vi "Master_DARPA_FUS2.vi"() -> ()   [LabVIEW 2021]
uses:
  Control 2.ctl
  Settings.ctl
  <vilib>/DAQmx/write.llb/DAQmx Write (Analog DBL 1Chan 1Samp).vi
  <vilib>/DAQmx/write.llb/DAQmx Write (Analog Wfm 1Chan NSamp).vi
  <vilib>/DAQmx/write.llb/DAQmx Write (Digital 1D U32 1Chan NSamp).vi
  <vilib>/DAQmx/read.llb/DAQmx Read (Counter DBL 1Chan 1Samp).vi
  <vilib>/DAQmx/create/channels.llb/DAQmx Create Channel (AO-Voltage-Basic).vi
  <vilib>/DAQmx/create/channels.llb/DAQmx Create Channel (CI-Count Edges).vi
  <vilib>/DAQmx/miscellaneous.llb/DAQmx Fill In Error Info.vi
  <vilib>/DAQmx/create/channels.llb/DAQmx Create Channel (DO-Digital Output).vi
  <vilib>/DAQmx/configure/timing.llb/DAQmx Timing (Sample Clock).vi
  <resource>/objmgr/daqmx.rc
panel:
  out "Trial End Signal":bool=TRUE
  in  "stop":bool
  in  "Blue Exposure Width [50-100] (ms)":T1=41.0 format="%#_9f"
  in  "Amber Start Time":T1=60.0 format="%#_9f"
  in  "Red Start (ms)":T1=120.0 format="%#_9f"
  in  "Red Exposure Width (ms)":T1=41.0 format="%#_9f"
  in  "Amber Exposure Width (ms)":T1=41.0 format="%#_9f"
  in  "base path":path=path "E:/DARPA/TUS-LSCI6"
  in  "Delay end (ms)":dbl=102.0
  out "Stimulation":bool=TRUE
  in  "AOM Voltage":dbl=0.085 format="%0.3f"
  out "String 7":string="AOM Settings"
  out "String 6":string="Stroke Settings"
  out "String 5":string="Intrinsic Imaging"
  in  "LED 625 nm":bool
  in  "LED 580 nm":bool
  out "Trial #":i32=6
  out "Frames acquired":dbl=9000.0 format="%0.2f"
  out "Number of Samples (Total)":dbl=18000.0
  out "Period (ms)":dbl=6.5
  out "String 4":string="Experimental Summary"
  out "String 3":string="Stimulation Control"
  out "String 2":string="Sequence Control"
  out "String":string="Trials Control"
  in  "# of stimulations":i32=112
  in  "Width of pulse (ms)":dbl=60.0
  in  "# of Sequences":dbl=750.0
  in  "Sampling Rate (Hz)":T1=100000.0 format="%#_9f"
  in  "Frames/Seq":i32=12
  in  "Exposure Width (ms)":T1=5.0 format="%#_9f"
  in  "Time Between (ms)":T2=1.5 format="%#_9f"
  in  "Pre-stimulus Time":dbl=30.0 format="%.6f"
  in  "Time b/w Trials (s)":dbl=5.0 caption="Delay Time (s)"
  in  "# Trials":i32=6
  in  "Time domain signal":T3(tab)=enum."Stimulation pulse"
  out "LSCI Sequence":cluster{i32, dbl, dbl[]}(graph)={0, 1e-05, array[18000 elements]}
  out "Red LED":cluster{i32, dbl, dbl[]}(graph)={0, 1e-05, array[18000 elements]}
  out "Amber LED":cluster{i32, dbl, dbl[]}(graph)={0, 1e-05, array[18000 elements]}
  out "Blue LED":cluster{i32, dbl, dbl[]}(graph)={0, 1e-05, array[18000 elements]}
  out "EMCCD":cluster{i32, dbl, dbl[]}(graph)={0, 1e-05, array[18000 elements]}
  out "Whisker Cam":cluster{i32, dbl, dbl[]}(graph)={0, 1e-05, array[18000 elements]}
  out "Whisker Stim":cluster{i32, dbl, dbl[]}(graph)={0, 1e-05, array[18000 elements]}
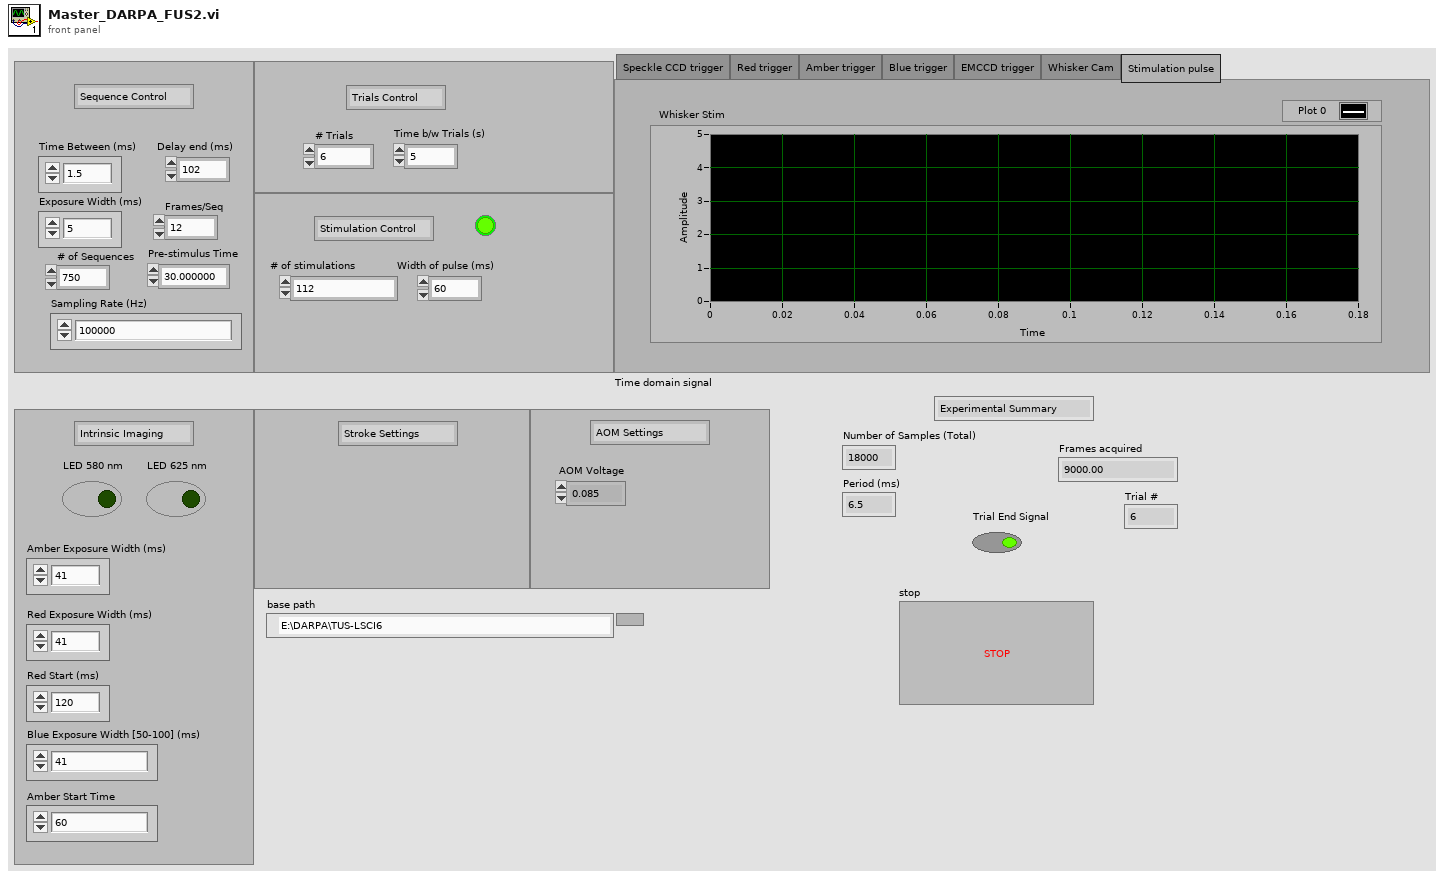
[diagram p1: front panel]
types:
  T1 = typedef "Settings.ctl" = dbl
  T2 = typedef "Control 2.ctl" = dbl
  T3 = enum32{"Speckle CCD trigger", "Red trigger", "Amber trigger", "Blue trigger", "EMCCD trigger", "Whisker Cam", "Stimulation pulse"}
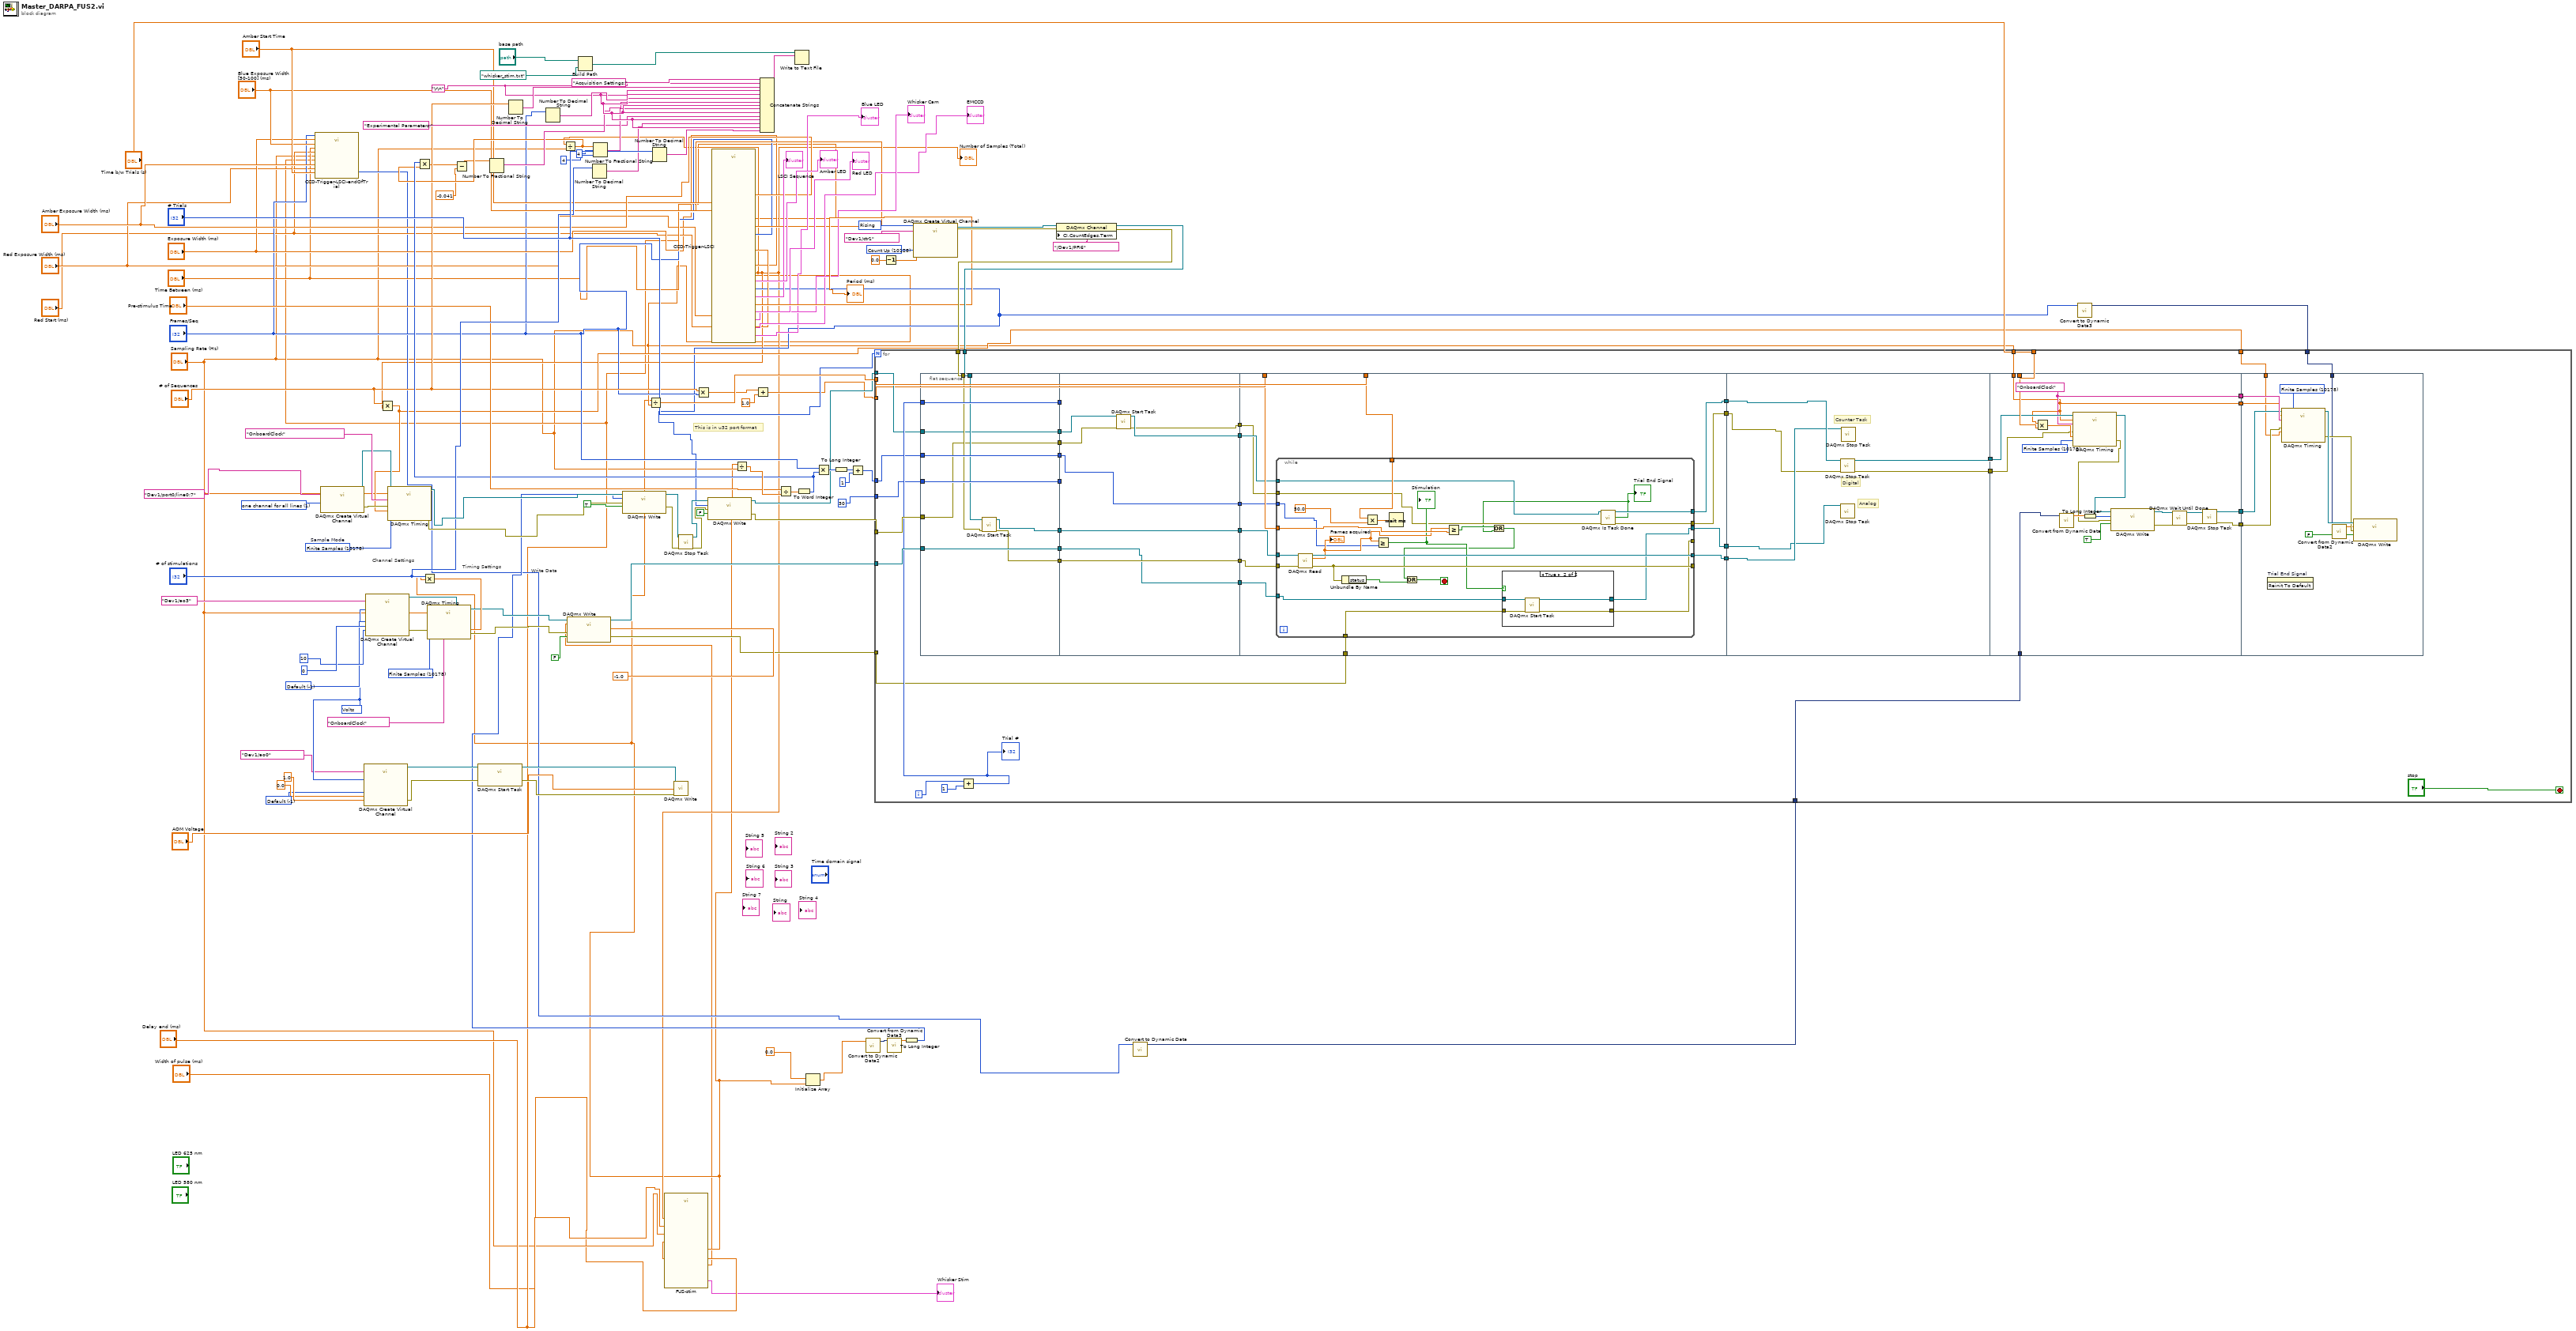
[diagram p0: block diagram]
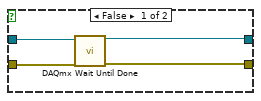
[diagram p2: hidden frame]
diagram:
  w64 = "\r\n"
  w74 = 1 items=["one channel for each line", "one channel for all lines"] ("line grouping")
  w89 = -1 items=["Default"=-1, "RSE"=10083, "Differential"=10106, "Pseudodifferential"=12529] ("output terminal configuration")
  w99 = 10280 items=["Rising"=10280, "Falling"=10171] ("edge")
  w103 = 10128 items=["Count Up"=10128, "Count Down"=10124, "Externally Controlled"=10326] ("count direction")
  w113 = 10178 items=["Finite Samples"=10178, "Continuous Samples"=10123] ("sample mode")
  w114 = -1 items=["Default"=-1, "RSE"=10083, "Differential"=10106, "Pseudodifferential"=12529] ("output terminal configuration")
  w91 = 10348 items=["Volts"=10348, "From Custom Scale"=10065] ("units")
  w119 = 10178 items=["Finite Samples"=10178, "Continuous Samples"=10123, "Hardware Timed Single Point"=12522]  # Sample Mode
  # "This is in u32 port format"
  # "Timing Settings"
  # "Write Data"
  # "Channel Settings"
  n1 = call "CCD-Trigger-LSCI-endOfTrial.vi"("Frames/Seq"="Frames/Seq", "Exposure Width (ms) in"="Exposure Width (ms)", "Blue Exposure Width [50-100] (ms)"="Blue Exposure Width [50-100] (ms)", "Time Between (ms)"="Time Between (ms)", "Red Start Time"="Red Start (ms)", "Sampling Rate"="Sampling Rate (Hz)", "Amber Start Time"="Amber Start Time", "Red Exposure Width [50-80] (ms)"="Red Exposure Width (ms)", "Amber Exposure Width [50-100] (ms)"="Amber Exposure Width (ms)", "Delay End (ms)"="Delay end (ms)") -> ("Array out"=w15:u32[])  [unwired: 1 in, 8 out]
  n2 = call-poly <vilib>:"DAQmx Create Virtual Channel.vi"("lines"=tag "Dev1/port0/line0:7", "line grouping"=w74) -> ("task out"=w81:refnum<k21>, "error out"=w107:errorcluster)  [unwired: 12 in]
  n3 = call-poly <vilib>:"DAQmx Create Virtual Channel.vi"("maximum value"=1.0, "minimum value"=0.0, "output terminal configuration"=w89, "physical channels"=tag "Dev1/ao0", "units"=w91) -> ("task out"=w87:refnum<k21>, "error out"=w86:errorcluster)  [unwired: 9 in]
  n4 = call-poly <vilib>:"DAQmx Create Virtual Channel.vi"("maximum value"=10, "minimum value"=0, "output terminal configuration"=w114, "physical channels"=tag "Dev1/ao3", "units"=w91) -> ("task out"=w111:refnum<k21>, "error out"=w112:errorcluster)  [unwired: 9 in]
  n5 = call <vilib>:"DAQmx Start Task.vi"("task/channels in"=w87, "error in"=w86) -> ("task out"=w85:refnum<k21>, "error out"=w84:errorcluster)  [unwired: 12 in]
  n6 = Number To Decimal String(number="# of Sequences") -> (decimal integer string=w66:string)  [unwired: 1 in]
  n7 = Number To Decimal String(number="Frames/Seq") -> (decimal integer string=w65:string)  [unwired: 1 in]
  n8 = Build Path(base path="base path", name or relative path=path "whisker_stim.txt" ("default name")) -> (appended path=w68:path)
  n9 = Number To Decimal String(number="# of stimulations") -> (decimal integer string=w59:string)  [unwired: 1 in]
  n10 = Number To Decimal String(number="# Trials") -> (decimal integer string=w63:string)  [unwired: 1 in]
  n11 = call-poly <vilib>:"DAQmx Write.vi"("task/channels in"=w85, "data"="AOM Voltage", "error in"=w84) -> ()  [unwired: 10 in, 3 out]
  n12 = Multiply(x="# of Sequences", y="Frames/Seq") -> (x*y=w18:dbl)
  n13 = call "CCD-Trigger-LSCI.vi"("Frames/Seq"="Frames/Seq", "Exposure Width (ms) in"="Exposure Width (ms)", "Blue Exposure Width [50-100] (ms)"="Blue Exposure Width [50-100] (ms)", "Time Between (ms)"="Time Between (ms)", "Red Start Time"="Red Start (ms)", "Sampling Rate"="Sampling Rate (Hz)", "Amber Start Time"="Amber Start Time", "Red Exposure Width [50-80] (ms)"="Red Exposure Width (ms)", "Amber Exposure Width [50-100] (ms)"="Amber Exposure Width (ms)", "Delay End (ms)"="Delay end (ms)") -> ("Blue LED"=→"Blue LED":cluster{i32, dbl, dbl[]}, "LSCI CCD"=→"LSCI Sequence":cluster{i32, dbl, dbl[]}, "Amber LED"=→"Amber LED":cluster{i32, dbl, dbl[]}, "Whisker Cam"=→"Whisker Cam":cluster{i32, dbl, dbl[]}, "EMCCD Trigger"=→"EMCCD":cluster{i32, dbl, dbl[]}, "Array out"=w12:u32[], "Period (ms)"=→"Period (ms)":dbl, "# Samples"=w7:T1, "Red LED"=→"Red LED":cluster{i32, dbl, dbl[]})  [unwired: 1 in]
  "Number of Samples (Total)" <- w7
  n14 = Multiply(x="# of Sequences", y=w7) -> (x*y=w13:T1)
  n15 = call-poly <vilib>:"DAQmx Timing.vi"("task/channels in"=w81, "sample mode"=w119, "samples per channel"=w13, "rate"="Sampling Rate (Hz)", "source"=tag "OnboardClock", "error in"=w107) -> ("task out"=w76:refnum<k21>, "error out"=w75:errorcluster)  [unwired: 8 in]
  n16 = Divide(x=w7, y="Sampling Rate (Hz)") -> (x/y=w48:T1)
  n17 = Number To Fractional String(number=w48, width (-)=i16 4, precision (6)=i16 4) -> (F-format string=w58:string)  [unwired: 1 in]
  n18 = call "FUS-stim.vi"("# Samples in"=w7, "Delay end (ms)"="Delay end (ms)", "Width of pulse (ms)"="Width of pulse (ms)", "Sampling Rate"="Sampling Rate (Hz)") -> ("Array 2"=w2:T1[], "# Samples out"=w3:T1, "Stimulation 2"=→"Whisker Stim":cluster{i32, dbl, dbl[]})  [unwired: 3 in, 2 out]
  n19 = Multiply(x="# of stimulations", y=w3) -> (x*y=w108:T1)
  n20 = call-poly <vilib>:"DAQmx Timing.vi"("task/channels in"=w111, "sample mode"=w113, "samples per channel"=w108, "rate"="Sampling Rate (Hz)", "source"=tag "OnboardClock", "error in"=w112) -> ("task out"=w78:refnum<k21>, "error out"=w77:errorcluster)  [unwired: 1 in, 7 out]
  n21 = call-poly <vilib>:"DAQmx Write.vi"("task/channels in"=w78, "auto start"=FALSE, "data"=w2, "timeout"=-1.0 ("Wirite Timeout"), "error in"=w77) -> ("task out"=w82:refnum<k21>, "error out"=w96:errorcluster)  [unwired: 9 out]
  n22 = Divide(x=w3, y="Sampling Rate (Hz)") -> (x/y=w95:T1)
  n23 = Divide(x=w3, y="Sampling Rate (Hz)") -> (x/y=w73:T1)
  n24 = Add(x=w18, y=1.0) -> (x+y=w16:dbl)
  n25 = Divide(x="Pre-stimulus Time", y=w73) -> (x/y=w52:T1)
  n26 = To Word Integer(number=w52) -> (16bit integer=w51:i16)
  n27 = Multiply(x=w51, y=w48) -> (x*y=w9:T1)
  n28 = Subtract(x=w9, y=-0.041) -> (x-y=w10:T1)
  n29 = Number To Fractional String(number=w10) -> (F-format string=w55:string)  [unwired: 3 in]
  n30 = Concatenate Strings("Acquisition Settings:" ("string"), w64, w66, w64, w65, w64, w55, w64, w58, w64, "Experimental Parameters:" ("string"), w64, w59, w64, w63) -> (w62:string)
  n31 = Write to Text File(file (use dialog)=w68, text=w62) -> ()  [unwired: 2 in, 3 out]
  n32 = Initialize Array(0.0 ("element"), w3) -> (w19:dbl[])
  n33 = Multiply(x="Frames/Seq", y=w51) -> (x*y=w53:i32)
  n34 = To Long Integer(number=w53) -> (32bit integer=w47:i32)
  n35 = Add(x=w47, y=1) -> (x+y=w45:i32)
  n36 = call "Convert to Dynamic Data2"("Array"=w19) -> ("Dynamic Data Type"=w37:dynamicdata)  [unwired: 3 in]
  n37 = Decrement(x=0.0) -> (x-1=w102:dbl)
  n38 = call "Convert from Dynamic Data3"("Dynamic Data Type"=w37) -> ("Array"=w36:dbl[])  [unwired: 3 in]
  n39 = To Long Integer(number=w36) -> (32bit integer=w35:i32[])
  n40 = call-poly <vilib>:"DAQmx Write.vi"("task/channels in"=w76, "auto start"=TRUE, "data"=w35, "error in"=w75) -> ("task out"=w31:refnum<k21>, "error out"=w29:errorcluster)  [unwired: 9 in, 1 out]
  n41 = call <vilib>:"DAQmx Stop Task.vi"("task/channels in"=w31, "error in"=w29) -> ("task out"=w30:refnum<k21>, "error out"=w28:errorcluster)  [unwired: 12 in]
  n42 = call-poly <vilib>:"DAQmx Write.vi"("task/channels in"=w30, "auto start"=FALSE, "data"=w12, "error in"=w28) -> ("task out"=w32:refnum<k21>, "error out"=w33:errorcluster)  [unwired: 9 in, 1 out]
  n43 = call-poly <vilib>:"DAQmx Create Virtual Channel.vi"("initial count"=w102, "count direction"=w103, "edge"=w99, "counter"=tag "Dev1/ctr1") -> ("task out"=w100:refnum<k21>, "error out"=w101:errorcluster)  [unwired: 10 in]
  n44 = property class="DAQmx Channel"(reference=w100, error in=w101, "CI.CountEdges.Term"=tag "/Dev1/PFI6") -> (reference out=w71:refnum<k21>, error out=w72:errorcluster)
  n45 = call "Convert to Dynamic Data"("Array"=w15) -> ("Dynamic Data Type"=w14:dynamicdata)  [unwired: 3 in]
  n46 = call "Convert to Dynamic Data3"("Array"=w12) -> ("Dynamic Data Type"=w11:dynamicdata)  [unwired: 3 in]
  n47 = for {
    N: "# Trials" -> [_]
    tunnel: w33 -> [w162]
    tunnel: w82 -> [w161]
    tunnel: w96 -> [w147]
    tunnel: w32 -> [w149]
    tunnel: w95 -> [w160]
    tunnel: w16 -> [w133]
    tunnel: "Time b/w Trials (s)" -> [w129]
    tunnel: u32 30 ("Frames Per Second") -> [w156]
    tunnel: w72 -> [w140]
    tunnel: w71 -> [w139]
    tunnel: w45 -> [w134]
    tunnel: w14 -> [w128]
    tunnel: w13 -> [w122]
    tunnel: w11 -> [w121]
    tunnel: "Sampling Rate (Hz)" -> [w120]
    i -> [w159]
    stop <- "stop" stop-if-true
    n48 = flat-sequence {
      tunnel: w156 -> [w170]
      tunnel: w157 -> [w171]
      tunnel: w161 -> [w172]
      tunnel: w162 -> [w163]
      tunnel: [w163] -> w153
      tunnel: [w172] -> w152
      tunnel: [w171] -> w151
      tunnel: [w170] -> w150
      tunnel: w149 -> [w164]
      tunnel: [w164] -> w148
      tunnel: [w169] -> w145
      tunnel: w134 -> [w169]
      tunnel: w140 -> [w168]
      tunnel: w139 -> [w167]
      tunnel: [w166] -> w137
      tunnel: [w165] -> w136
      tunnel: w153 -> [w176]
      tunnel: w152 -> [w173]
      tunnel: w151 -> [_]
      tunnel: w150 -> [_]
      tunnel: w148 -> [w177]
      tunnel: [w175] -> w144
      tunnel: [w173] -> w143
      tunnel: [w180] -> w142
      tunnel: w145 -> [w180]
      tunnel: [w179] -> w138
      tunnel: w137 -> [w179]
      tunnel: w136 -> [w178]
      tunnel: [w178] -> w135
      tunnel: [w174] -> w132
      tunnel: w160 -> [w193]
      tunnel: w133 -> [w192]
      tunnel: [w191] -> w155
      tunnel: [w182] -> w154
      tunnel: w144 -> [w184]
      tunnel: w147 -> [w190]
      tunnel: w143 -> [w189]
      tunnel: [w188] -> w146
      tunnel: w142 -> [w187]
      tunnel: [w181] -> w141
      tunnel: w138 -> [w186]
      tunnel: w135 -> [w185]
      tunnel: w132 -> [w183]
      tunnel: w155 -> [w230]
      tunnel: w154 -> [w231]
      tunnel: w146 -> [w229]
      tunnel: w141 -> [w228]
      tunnel: [w227] -> w130
      tunnel: [w226] -> w127
      tunnel: w130 -> [w247]
      tunnel: w129 -> [w248]
      tunnel: w128 -> [w244]
      tunnel: w127 -> [w246]
      tunnel: [w233] -> w126
      tunnel: [w239] -> w125
      tunnel: [w236] -> w124
      tunnel: [w232] -> w123
      tunnel: w120 -> [w236]
      tunnel: w126 -> [w259]
      tunnel: w125 -> [w261]
      tunnel: w124 -> [w260]
      tunnel: w123 -> [w258]
      tunnel: w122 -> [w257]
      tunnel: w121 -> [w253]
      frame #0 {
        n49 = call <vilib>:"DAQmx Start Task.vi"("task/channels in"=w167, "error in"=w168) -> ("task out"=w166:refnum<k21>, "error out"=w165:errorcluster)  [unwired: 12 in]
      }
      frame #1 {
        n50 = call <vilib>:"DAQmx Start Task.vi"("task/channels in"=w177, "error in"=w176) -> ("task out"=w175:refnum<k21>, "error out"=w174:errorcluster)  [unwired: 12 out]
      }
      frame #2 {
        n51 = while {
          tunnel: w186 -> [w217]
          tunnel: w185 -> [w216]
          tunnel: [w215] -> w191
          tunnel: [w214] -> _
          tunnel: w193 -> [w213]
          tunnel: w192 -> [w206]
          tunnel: w190 -> [w209]
          tunnel: w189 -> [w210]
          tunnel: [w207] -> w188
          tunnel: [w208] -> _
          tunnel: w187 -> [w202]
          tunnel: w184 -> [w200]
          tunnel: w183 -> [w199]
          tunnel: [w198] -> w182
          tunnel: [w197] -> w181
          stop <- w203 stop-if-true
          n52 = call-poly <vilib>:"DAQmx Read.vi"("task/channels in"=w217, "error in"=w216) -> ("task out"=w215:refnum<k21>, "data"=w205:dbl, "error out"=w214:errorcluster)  [unwired: 11 in]
          "Frames acquired" <- w205
          n53 = Unbundle By Name(w214) -> ("status"=w204:bool)
          n54 = Multiply(x=w213, y=T1 50.0) -> (x*y=w212:T1)
          n55 = Greater Or Equal?(x=w205, y=w202) -> (x >= y?=w201:bool)
          "Stimulation" <- w201
          n56 = Wait (ms)(milliseconds to wait=w212) -> ()  [unwired: 1 out]
          n57 = Greater Or Equal?(x=w205, y=w206) -> (x >= y?=w196:bool)
          n58 = case shown="True" w201 {
            tunnel: w210 -> [w221 w225]
            tunnel: w209 -> [w220 w224]
            tunnel: [w218 w223] -> w208
            tunnel: [w219 w222] -> w207
            frame False {
              n59 = call <vilib>:"DAQmx Wait Until Done.vi"("task/channels in"=w221, "error in"=w220) -> ("task out"=w219:refnum<k21>, "error out"=w218:errorcluster)  [unwired: 12 in]
            }
            frame True {
              n60 = call <vilib>:"DAQmx Start Task.vi"("task/channels in"=w225, "error in"=w224) -> ("task out"=w222:refnum<k21>, "error out"=w223:errorcluster)  [unwired: 12 out]
            }
          }
          n61 = call <vilib>:"DAQmx Is Task Done.vi"("task/channels in"=w200, "error in"=w199) -> ("task out"=w198:refnum<k21>, "task done?"=w195:bool, "error out"=w197:errorcluster)  [unwired: 11 in]
          "Trial End Signal" <- w195
          n62 = Or(x=w196, y=w195) -> (x .or. y?=w194:bool)
          n63 = Or(x=w194, y=w204) -> (x .or. y?=w203:bool)
        }
      }
      frame #3 {
        # "Analog"
        # "Digital"
        # "Counter Task"
        n64 = call <vilib>:"DAQmx Stop Task.vi"("task/channels in"=w231, "error in"=w228) -> ("task out"=w227:refnum<k21>, "error out"=w226:errorcluster)  [unwired: 12 in]
        n65 = call <vilib>:"DAQmx Stop Task.vi"("task/channels in"=w229) -> ()  [unwired: 13 in, 2 out]
        n66 = call <vilib>:"DAQmx Stop Task.vi"("task/channels in"=w230) -> ()  [unwired: 13 in, 2 out]
      }
      frame #4 {
        w239 = tag "OnboardClock" ("source")
        w250 = 10178 items=["Finite Samples"=10178, "Continuous Samples"=10123, "Hardware Timed Single Point"=12522] ("sample mode")
        n67 = Multiply(x=w236, y=w248) -> (x*y=w249:T1)
        n68 = call "Convert from Dynamic Data"("Dynamic Data Type"=w244) -> ("Array"=w243:dbl[])  [unwired: 3 in]
        n69 = call-poly <vilib>:"DAQmx Timing.vi"("task/channels in"=w247, "sample mode"=w250, "samples per channel"=w249, "rate"=w236, "source"=w239, "error in"=w246) -> ("task out"=w245:refnum<k21>, "error out"=w241:errorcluster)  [unwired: 8 in]
        n70 = To Long Integer(number=w243) -> (32bit integer=w242:i32[])
        n71 = call-poly <vilib>:"DAQmx Write.vi"("task/channels in"=w245, "auto start"=TRUE, "data"=w242, "error in"=w241) -> ("task out"=w238:refnum<k21>, "error out"=w237:errorcluster)  [unwired: 9 in, 1 out]
        n72 = call <vilib>:"DAQmx Wait Until Done.vi"("task/channels in"=w238, "error in"=w237) -> ("task out"=w235:refnum<k21>, "error out"=w234:errorcluster)  [unwired: 12 in]
        n73 = call <vilib>:"DAQmx Stop Task.vi"("task/channels in"=w235, "error in"=w234) -> ("task out"=w233:refnum<k21>, "error out"=w232:errorcluster)  [unwired: 12 in]
      }
      frame #5 {
        w256 = 10178 items=["Finite Samples"=10178, "Continuous Samples"=10123, "Hardware Timed Single Point"=12522] ("sample mode")
        n74 = invoke on="Trial End Signal" class="Bool (strict)" method="Reinit To Default"() -> ()  [unwired: 3 in, 3 out]
        n75 = call-poly <vilib>:"DAQmx Timing.vi"("task/channels in"=w259, "sample mode"=w256, "samples per channel"=w257, "rate"=w260, "source"=w261, "error in"=w258) -> ("task out"=w255:refnum<k21>, "error out"=w254:errorcluster)  [unwired: 8 in]
        n76 = call "Convert from Dynamic Data2"("Dynamic Data Type"=w253) -> ("Array"=w252:dbl[])  [unwired: 3 in]
        n77 = call-poly <vilib>:"DAQmx Write.vi"("task/channels in"=w255, "auto start"=FALSE, "data"=w252, "error in"=w254) -> ()  [unwired: 9 in, 3 out]
      }
    }
    n78 = Add(x=w159, y=1) -> (x+y=w157:i32)
    "Trial #" <- w157
  }
